vi "Log Temp.vi"(8 "error in (no error)":errorcluster, 10 "Status string":string, 11 "Temperature Controller in":refnum<class "Temperature Controller.lvclass">) -> (0 "error out":errorcluster, 3 "Temperature Controller out":refnum<class "Temperature Controller.lvclass">)   [LabVIEW 2023, in "Temperature Controller.lvclass"]
uses:
  Temperature Controller.lvclass
  Global/File Locations.vi
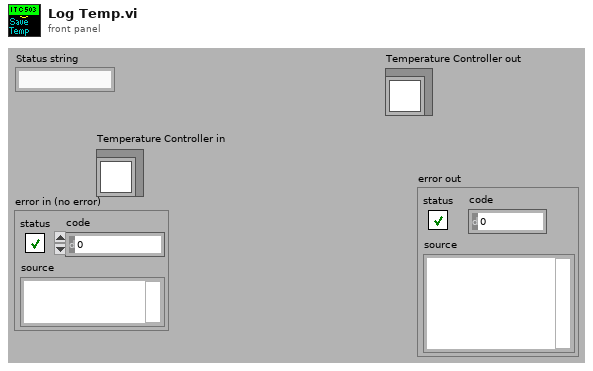
[diagram p1: front panel]
types:
  T1 = enum16{"open", "open or create", "create or replace", "create", "open (read only)"}
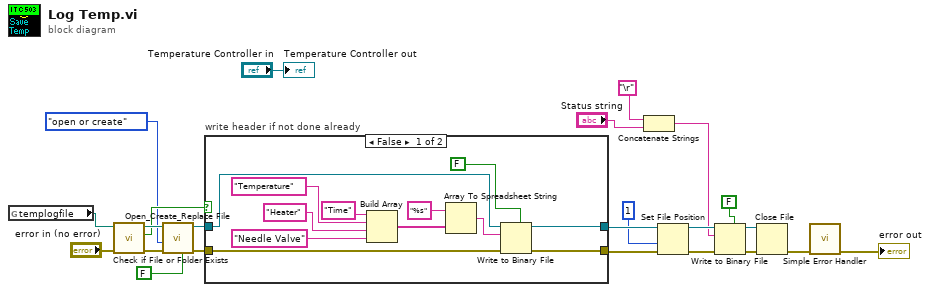
[diagram p0: block diagram]
diagram:
  n1 = global read "File Locations.vi" "templogfile"() -> (w4:path)
  n2 = call <vilib>:"Check if File or Folder Exists.vi"("error in (no error)"="error in (no error)", "path"=w4) -> ("error out"=w15:errorcluster, "file or folder exists?"=w22:bool, "dup path"=w23:path)  [unwired: 7 out]
  n3 = call <vilib>:"Open_Create_Replace File.vi"("advisory dialog? (display:T)"=FALSE, "error in (no error)"=w15, "function (open:0)"=T1."open or create", "file path"=w23) -> ("error out"=w20:errorcluster, "refnum"=w21:refnum<file>)  [unwired: 3 in, 3 out]
  n4 = case "write header if not done already" shown="False" w22 {
    tunnel: w21 -> [w35 w37]
    tunnel: w20 -> [w34 w36]
    tunnel: [w33 w36] -> w18
    tunnel: [w28 w37] -> w19
    frame False {
      n5 = Build Array("Time", "Temperature", "Heater", "Needle Valve") -> (w26:string[])
      n6 = Array To Spreadsheet String(array=w26, 3:"%s" ("format string")) -> (spreadsheet string=w25:string)  [unwired: 1 in]
      n7 = Write to Binary File(file (use dialog)=w35, data=w25, error in=w34, 5:FALSE ("prepend array or string size? (T)")) -> (refnum out=w28:refnum<file>, error out=w33:errorcluster)  [unwired: 3 out]
    }
    frame True {
    }
  }
  n8 = Concatenate Strings("\r", "Status string") -> (w5:string)
  n9 = Set File Position(refnum=w19, from (0:start)=1, error in=w18) -> (refnum out=w14:refnum<file>, error out=w13:errorcluster)  [unwired: 1 out]
  n10 = Write to Binary File(file (use dialog)=w14, data=w5, error in=w13, 5:FALSE ("prepend array or string size? (T)")) -> (refnum out=w17:refnum<file>, error out=w16:errorcluster)  [unwired: 3 out]
  n11 = Close File(refnum=w17, error in=w16) -> (error out=w2:errorcluster)  [unwired: 1 out]
  n12 = call <vilib>:"Simple Error Handler.vi"("error in (no error)"=w2) -> ("error out"=→"error out":errorcluster)  [unwired: 4 in, 4 out]
  "Temperature Controller out" <- "Temperature Controller in"
